vi "SetState.vi"(8 "error in (no error)":errorcluster, 9 "State":T1=enum."有硬幣", 11 "GumballMachine in":refnum<class "GumballMachine.lvclass">) -> (0 "error out":errorcluster, 3 "GumballMachine out":refnum<class "GumballMachine.lvclass">)   [LabVIEW 2013, in "GumballMachine.lvclass"]
uses:
  GumballMachine.lvclass
  StateMark.ctl
  GumballMachine.lvclass/GumballMachine.ctl
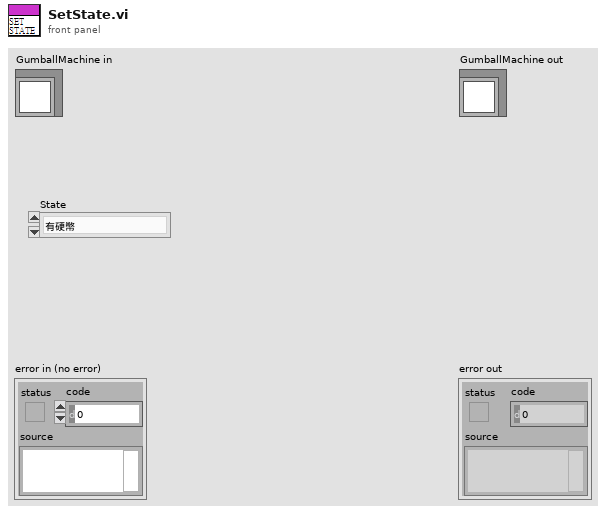
[diagram p1: front panel]
types:
  T1 = typedef "StateMark.ctl" = enum16{"沒有硬幣", "有硬幣", "賣出糖果", "糖果賣完", "NoChange"}
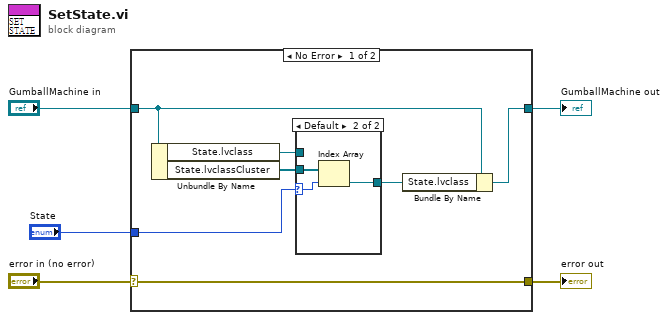
[diagram p0: block diagram]
diagram:
  n1 = case shown="No Error" "error in (no error)" {
    selector: "error in (no error)" -> [w12 w18]
    tunnel: [w12 w18] -> w4
    tunnel: [w8 w17] -> w2
    tunnel: "GumballMachine in" -> [w9 w17]
    tunnel: "State" -> [w7 _]
    frame No Error {
      n2 = Unbundle By Name(w9) -> ("State.lvclass"=w6:refnum<class "State.lvclass">, "State.lvclassCluster"=w11:refnum<class "State.lvclass">[])
      n3 = case shown="Default" w7 {
        selector: w7 -> [_ w14]
        tunnel: w11 -> [_ w16]
        tunnel: [w13 w15] -> w10
        tunnel: w6 -> [w13 _]
        frame "NoChange" {
        }
        frame Default {
          n4 = Index Array(array=w16, index=w14) -> (element=w15:refnum<class "State.lvclass">)
        }
      }
      n5 = Bundle By Name(cluster=w9, "State.lvclass"=w10) -> (w8:refnum<class "GumballMachine.lvclass">)
    }
    frame Error {
    }
  }
  "error out" <- w4
  "GumballMachine out" <- w2
